vi "instrument.vi"(0 "Commands":string, 11 "error in (no error)":errorcluster) -> (4 "Output":string, 15 "error out":errorcluster)   [LabVIEW 2023]
doc: "This is an instrument to set and get data."
uses:
  <vilib>/Utility/config.llb/Read Key (Double).vi
  <vilib>/regexp/Match Regular Expression.xnode
  <vilib>/Utility/config.llb/NI_LVConfig.lvlib
panel:
  # "Notes:\n    - To configure the error percentge of the data being \n       saved by the instrument,\n     1) Open the cinfig.vi present along with the instrument.vi\n     2) The first line must be \"[0]\" , add if not present already.\n     3) In the next line \"error_% = 10\" to set the error value of 10%\n     4) Change the value as required."
  # "code - 85 source with a non double argument\ncode 19 read key was not double\ncode 5001 invalid parameter. (VOLT?CURR)\ncode 5003 invalid operation (SOUR/MEAS)\ncode 5005 Invalid read format\ncode 5007 Invalid write format"
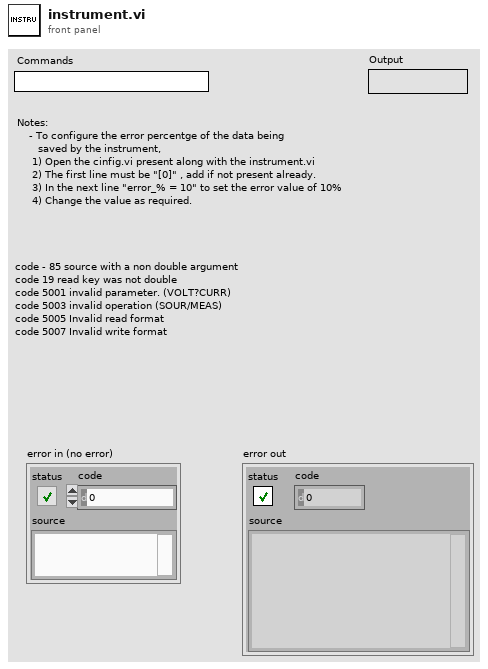
[diagram p1: front panel]
types:
  T1 = typedef "NI_LVConfig.lvlib/Config Data RefNum.ctl" = refnum<k1>
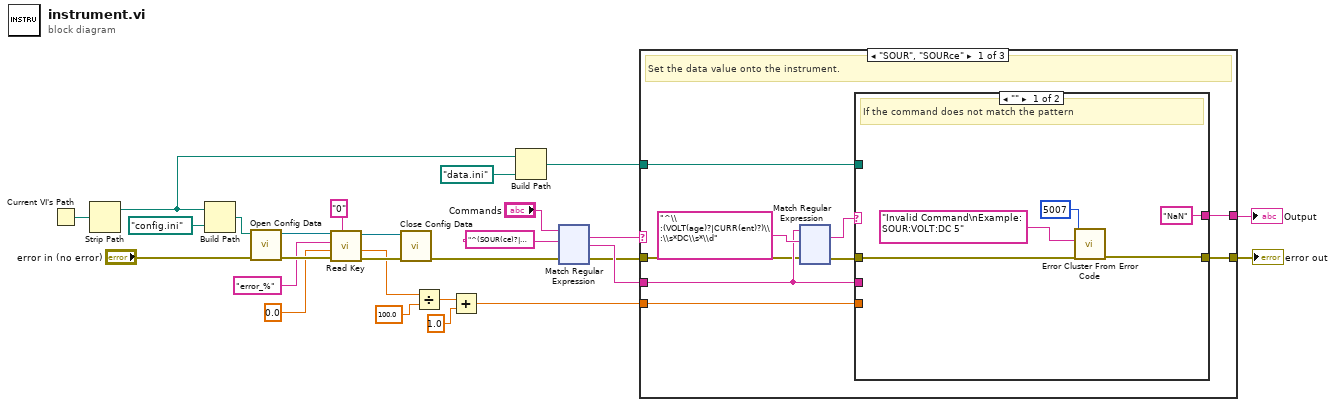
[diagram p0: block diagram]
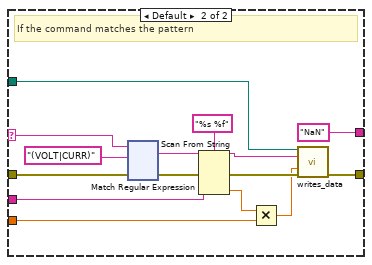
[diagram p2: hidden frame]
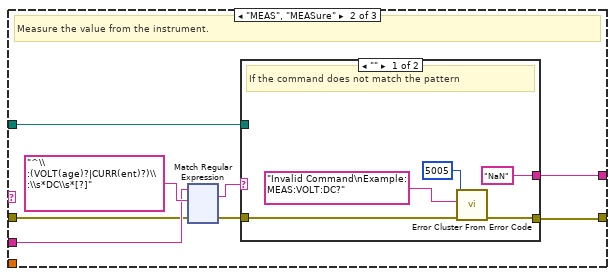
[diagram p3: hidden frame]
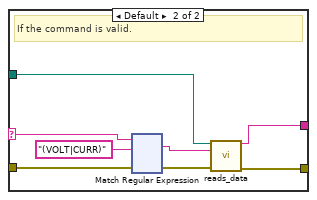
[diagram p4: hidden frame]
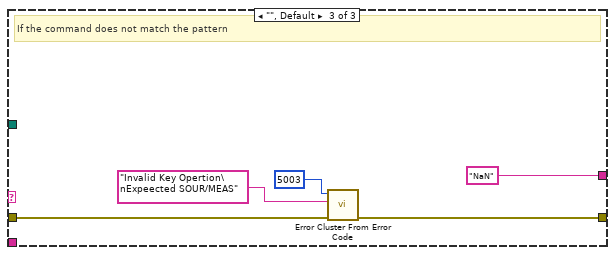
[diagram p5: hidden frame]
diagram:
  n1 = Current VI's Path() -> (path=w22:path)
  n2 = Strip Path(path=w22) -> (stripped path=w3:path)  [unwired: 1 out]
  n3 = Build Path(base path=w3, name or relative path=path "config.ini") -> (appended path=w20:path)
  n4 = call <vilib>:"Open Config Data.vi"("error in (no error)"="error in (no error)", "configuration file path"=w20) -> ("error out"=w17:errorcluster, "refnum"=w18:T1)  [unwired: 7 in, 1 out]
  n5 = call-poly <vilib>:"Read Key.vi"("section"="0", "error in (no error)"=w17, "default value"=0.0, "key"="error_%", "refnum"=w18) -> ("error out"=w16:errorcluster, "value"=w11:dbl, "refnum out"=w12:T1)  [unwired: 3 in, 1 out]
  n6 = call <vilib>:"Close Config Data.vi"("error in (no error)"=w16, "refnum"=w12) -> ("error out"=w2:errorcluster)  [unwired: 8 in, 1 out]
  n7 = Divide(x=w11, y=100.0) -> (x/y=w8:dbl)
  n8 = Add(x=w8, y=1.0) -> (x+y=w9:dbl)
  n9 = Build Path(base path=w3, name or relative path=path "data.ini") -> (appended path=w5:path)
  n10 = xnode "Match Regular Expression"("input string"="Commands", "regular expression"="^(SOUR(ce)?|MEAS(ure)?)", "error in"=w2) -> ("whole match"=w26:string, "after match"=w25:string, "error out"=w1:errorcluster)  [unwired: 3 in, 2 out]
  n11 = case shown="\"SOUR\", \"SOURce\"" w26 {
    tunnel: w5 -> [w36 w293 _]
    tunnel: w1 -> [w29 w291 w549]
    tunnel: w25 -> [w32 w295 _]
    tunnel: [w33 w294 w548] -> w24
    tunnel: [w31 w292 "NaN"] -> w23
    tunnel: w9 -> [w30 _ _]
    frame "SOUR", "SOURce" {
      # "Set the data value onto the instrument."
      n12 = xnode "Match Regular Expression"("input string"=w32, "regular expression"="^\\:(VOLT(age)?|CURR(ent)?)\\:\\s*DC\\s*\\d", "error in"=w29) -> ("whole match"=w35:string, "error out"=w28:errorcluster)  [unwired: 3 in, 3 out]
      n13 = case shown="\"\"" w35 {
        selector: w35 -> [_ w54]
        tunnel: w36 -> [_ w55]
        tunnel: [w37 w51] -> w33
        tunnel: w28 -> [w38 w43]
        tunnel: w32 -> [_ w48]
        tunnel: ["NaN" "NaN"] -> w31
        tunnel: w30 -> [_ w44]
        frame "" {
          # "If the command does not match the pattern"
          n14 = call <vilib>:"Error Cluster From Error Code.vi"("error in (no error)"=w38, "error message (\"\")"="Invalid Command\nExample: SOUR:VOLT:DC 5" ("error message (\"\")"), "error code (0)"=5007) -> ("error out"=w37:errorcluster)  [unwired: 6 in]
        }
        frame Default {
          # "If the command matches the pattern"
          n15 = xnode "Match Regular Expression"("input string"=w54, "regular expression"="(VOLT|CURR)", "error in"=w43) -> ("whole match"=w49:string, "error out"=w42:errorcluster)  [unwired: 3 in, 3 out]
          n16 = Scan From String(format string="%s %f", input string=w48, error in=w42) -> (error out=w50:errorcluster, output 2=w45:dbl)  [unwired: 4 in, 2 out]
          n17 = Multiply(x=w45, y=w44) -> (x*y=w46:dbl)
          n18 = call "writes_data.vi"("Path"=w55, "Key"=w49, "Value"=w46, "error in (no error)"=w50) -> ("error out"=w51:errorcluster)  [unwired: 11 in]
        }
      }
    }
    frame "MEAS", "MEASure" {
      # "Measure the value from the instrument."
      n19 = xnode "Match Regular Expression"("input string"=w295, "regular expression"="^\\:(VOLT(age)?|CURR(ent)?)\\:\\s*DC\\s*[?]", "error in"=w291) -> ("whole match"=w297:string, "error out"=w290:errorcluster)  [unwired: 3 in, 3 out]
      n20 = case shown="\"\"" w297 {
        selector: w297 -> [_ w310]
        tunnel: [w300 w308] -> w294
        tunnel: w290 -> [w301 w304]
        tunnel: w293 -> [_ w306]
        tunnel: ["NaN" ("Value") w305] -> w292
        frame "" {
          # "If the command does not match the pattern"
          n21 = call <vilib>:"Error Cluster From Error Code.vi"("error in (no error)"=w301, "error message (\"\")"="Invalid Command\nExample: MEAS:VOLT:DC?" ("error message (\"\")"), "error code (0)"=5005) -> ("error out"=w300:errorcluster)  [unwired: 6 in]
        }
        frame Default {
          # "If the command is valid."
          n22 = xnode "Match Regular Expression"("input string"=w310, "regular expression"="(VOLT|CURR)", "error in"=w304) -> ("whole match"=w307:string, "error out"=w303:errorcluster)  [unwired: 3 in, 3 out]
          n23 = call "reads_data.vi"("Path"=w306, "Key"=w307, "error in (no error)"=w303) -> ("Value"=w305:string, "error out"=w308:errorcluster)  [unwired: 11 in]
        }
      }
    }
    frame "", Default {
      # "If the command does not match the pattern"
      n24 = call <vilib>:"Error Cluster From Error Code.vi"("error in (no error)"=w549, "error message (\"\")"="Invalid Key Opertion\nExpeected SOUR/MEAS" ("error message (\"\")"), "error code (0)"=5003) -> ("error out"=w548:errorcluster)  [unwired: 6 in]
    }
  }
  "error out" <- w24
  "Output" <- w23
